vi "Enable_Disable Single Control.vi"(8 "error in (no error)":errorcluster, 9 "Enable (T)":bool, 10 "Control Name":string, 11 "Rename in":refnum<class "Rename.lvclass">) -> (0 "error out":errorcluster, 3 "Rename out":refnum<class "Rename.lvclass">)   [LabVIEW 2015, in "Generic Module Library.lvlib" / "Template G_Module.lvlib" / "Rename.lvclass"]
uses:
  Rename.lvclass
  Private API/Module Control Manager/Control_Mgr_Class/Controls_Mgr.lvclass
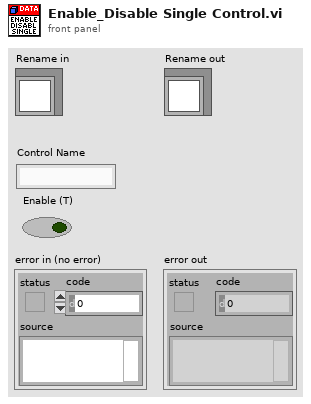
[diagram p1: front panel]
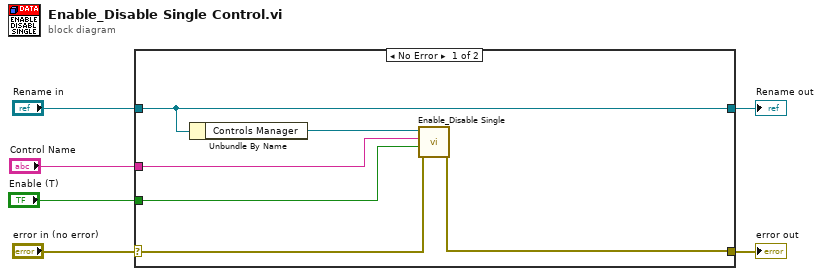
[diagram p0: block diagram]
diagram:
  n1 = case shown="No Error" "error in (no error)" {
    selector: "error in (no error)" -> [w8 w14]
    tunnel: [w7 w14] -> w5
    tunnel: [w12 w13] -> w3
    tunnel: "Rename in" -> [w12 w13]
    tunnel: "Control Name" -> [w10 _]
    tunnel: "Enable (T)" -> [w9 _]
    frame No Error {
      n2 = Unbundle By Name(w12) -> ("Controls Manager"=w11:refnum<class "Controls_Mgr.lvclass">)
      n3 = call "Enable_Disable Single.vi"("error in (no error)"=w8, "Enable (T)"=w9, "Control Name"=w10, "Controls_Mgr in"=w11) -> ("error out"=w7:errorcluster)  [unwired: 6 in, 1 out]
    }
    frame Error {
    }
  }
  "error out" <- w5
  "Rename out" <- w3
